vi "Continuous Buffered Acquisition.vi"() -> ()   [LabVIEW 2009]
uses:
  <vilib>/DAQmx/configure/timing.llb/DAQmx Timing (Sample Clock).vi
  <vilib>/DAQmx/create/channels.llb/DAQmx Create Channel (AI-Voltage-Basic).vi
  <vilib>/DAQmx/read.llb/DAQmx Read (Analog Wfm 1Chan NSamp).vi
  Program Files/National Instruments/LabVIEW 2009/resource/objmgr/daqmx.rc
panel:
  out "AvailSampPerChan":u32
  in  "physical channels":tag
  in  "rate":dbl=1000.0 format="%0.2f"
  in  "stop":bool
  out "data":waveform(dbl)(graph)
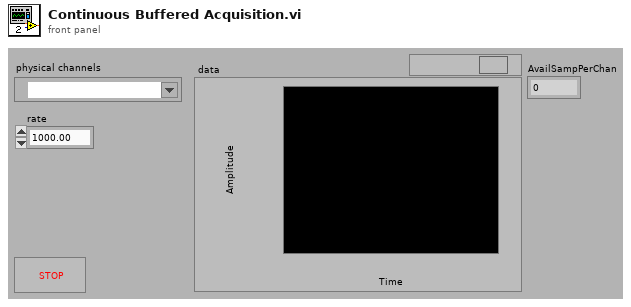
[diagram p1: front panel]
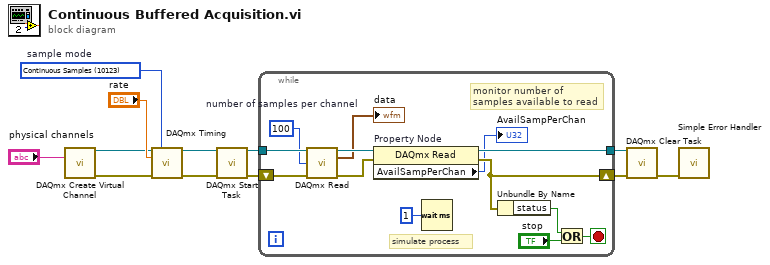
[diagram p0: block diagram]
diagram:
  w11 = 10123 items=["Finite Samples"=10178, "Continuous Samples"=10123, "Hardware Timed Single Point"=12522]  # sample mode
  n1 = call-poly <vilib>:"DAQmx Create Virtual Channel.vi"("physical channels"="physical channels") -> ("task out"=w9:refnum<k21>, "error out"=w2:errorcluster)  [unwired: 13 in]
  n2 = call-poly <vilib>:"DAQmx Timing.vi"("task/channels in"=w9, "sample mode"=w11, "rate"="rate", "error in"=w2) -> ("task out"=w8:refnum<k21>, "error out"=w3:errorcluster)  [unwired: 10 in]
  n3 = call <vilib>:"DAQmx Start Task.vi"("task/channels in"=w8, "error in"=w3) -> ("task out"=w7:refnum<k21>, "error out"=w4:errorcluster)  [unwired: 12 in]
  n4 = while {
    tunnel: [w17] -> w6
    tunnel: w7 -> [w24]
    shift-right: [w15] -> w1
    shift-left: w4 -> [w25]
    stop <- w23 stop-if-true
    w21 = 100  # number of samples per channel
    # "monitor number of samples available to read"
    # "simulate process"
    n5 = call-poly <vilib>:"DAQmx Read.vi"("task/channels in"=w24, "number of samples per channel"=w21, "error in"=w25) -> ("task out"=w18:refnum<k21>, "data"=→"data":waveform(dbl), "error out"=w16:errorcluster)  [unwired: 10 in]
    n6 = property on="Property Node" class="DAQmx Read"(reference=w18, error in=w16) -> (reference out=w17:refnum<k21>, error out=w15:errorcluster, "AvailSampPerChan"=→"AvailSampPerChan":u32)
    n7 = Wait (ms)(milliseconds to wait=u32 1) -> ()  [unwired: 1 out]
    n8 = Unbundle By Name "Unbundle By Name"(w15) -> ("status"=w20:bool)
    n9 = Or(x=w20, y="stop") -> (x .or. y?=w23:bool)
  }
  n10 = call <vilib>:"DAQmx Clear Task.vi"("task in"=w6, "error in"=w1) -> ("error out"=w5:errorcluster)  [unwired: 13 in]
  n11 = call <vilib>:"Simple Error Handler.vi"("error in (no error)"=w5) -> ()  [unwired: 4 in, 5 out]
